vi "SmartSEM Remote API save FIB probe table.vi"(8 "error in":errorcluster, 10 "FIB Probe":string(combo), 11 "ActiveX Container":refnum<k7>(container)) -> (0 "error out":errorcluster, 3 "reference out":refnum<k7>)   [LabVIEW 2018]
uses:
  <vilib>/Utility/file.llb/Write To Spreadsheet File (string).vi
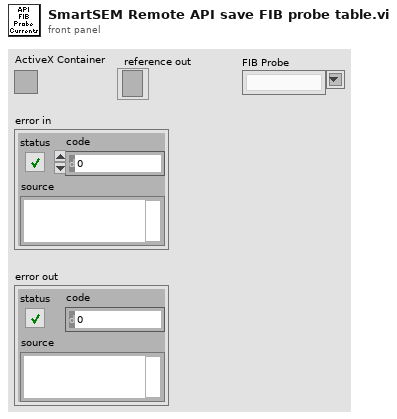
[diagram p1: front panel]
types:
  T1 = cluster{"FIB mode":u8, "FIB focus":sgl, "FIB probe current":sgl, "FIB emission current":sgl, "FIB rotation":sgl, "FIB aperture X":sgl, "FIB aperture Y":sgl, "FIB stig X":sgl, "FIB stig Y":sgl, "FIB beam shift X":sgl, "FIB beam shift Y":sgl}
  T2 = cluster{"Filament (A)":sgl, "Accelerator Target (V)":sgl, "Accelerator Actual (V)":sgl, "Extrator Target (V)":sgl, "Extrator Actual (V)":sgl, "Emission Target (uA)":sgl, "Emission Actual (uA)":sgl, "Suppressor (V)":sgl, "Faraday I (nA)":sgl, "Lens1 Target (V)":sgl, "Lens1 Actual (V)":sgl, "Lens2 Target (V)":sgl, "Lens2 Actual (V)":sgl, "Gun Vac (Torr)":sgl, "Column Vac (Torr)":sgl, "Tip Lifetime (uAhr)":sgl}
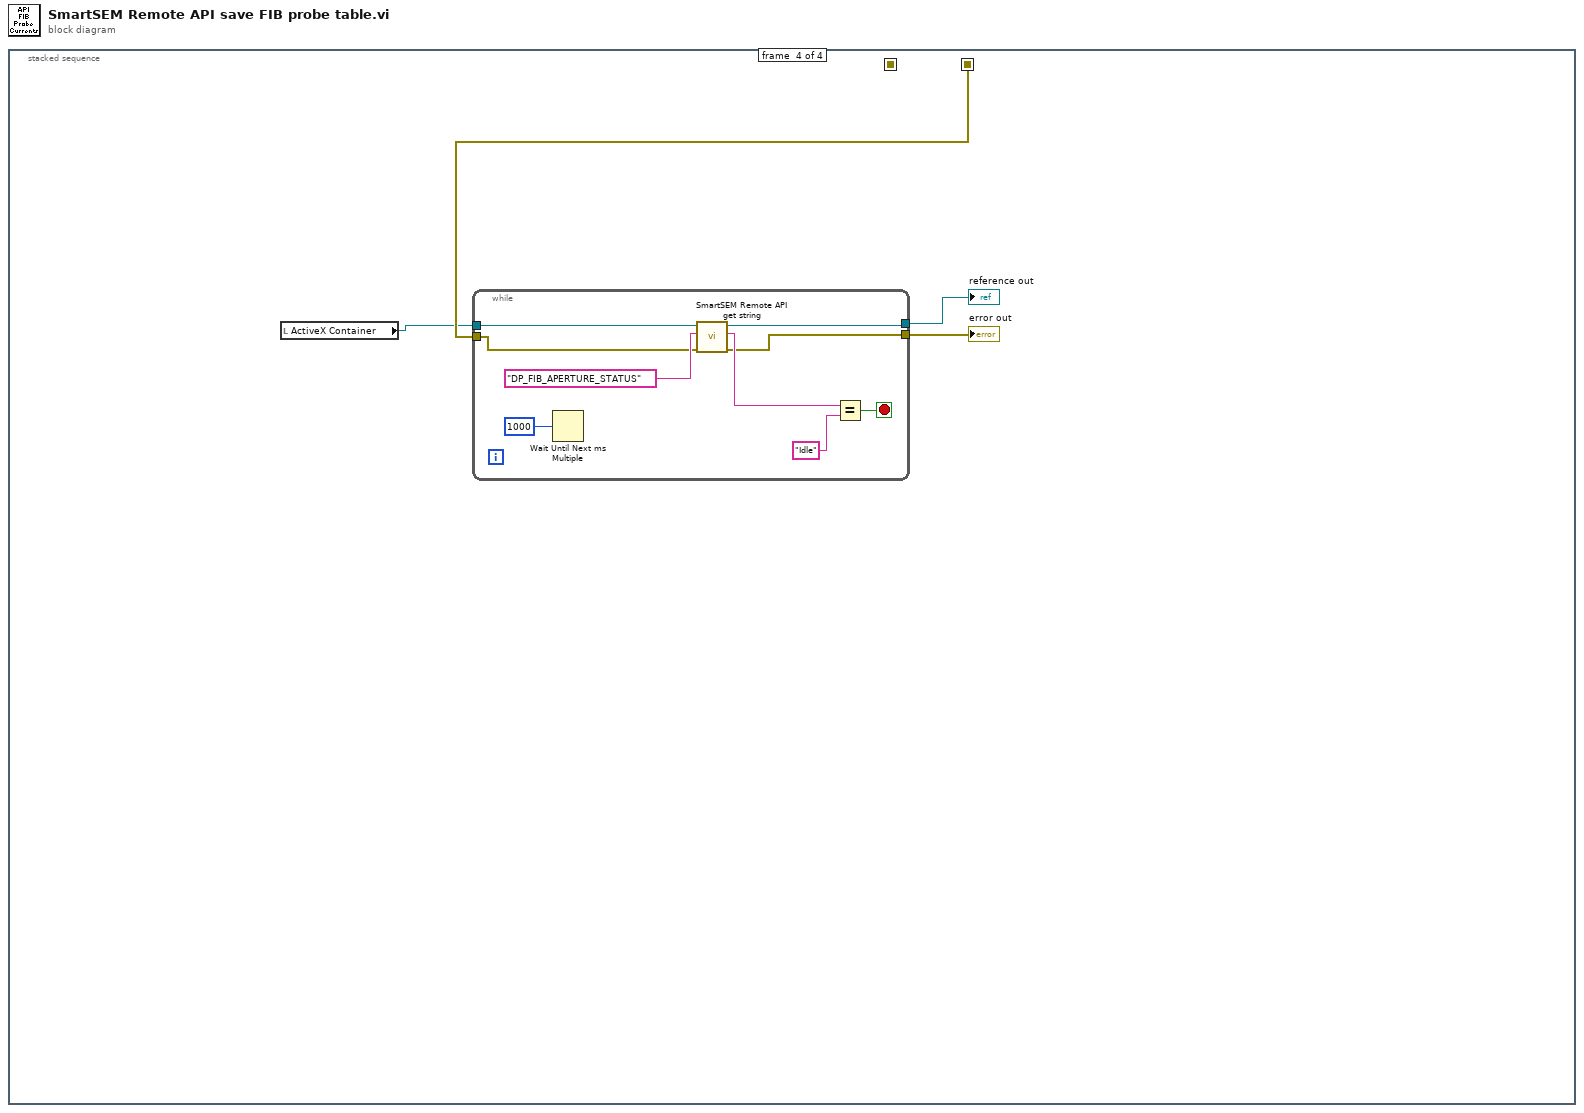
[diagram p0: block diagram]
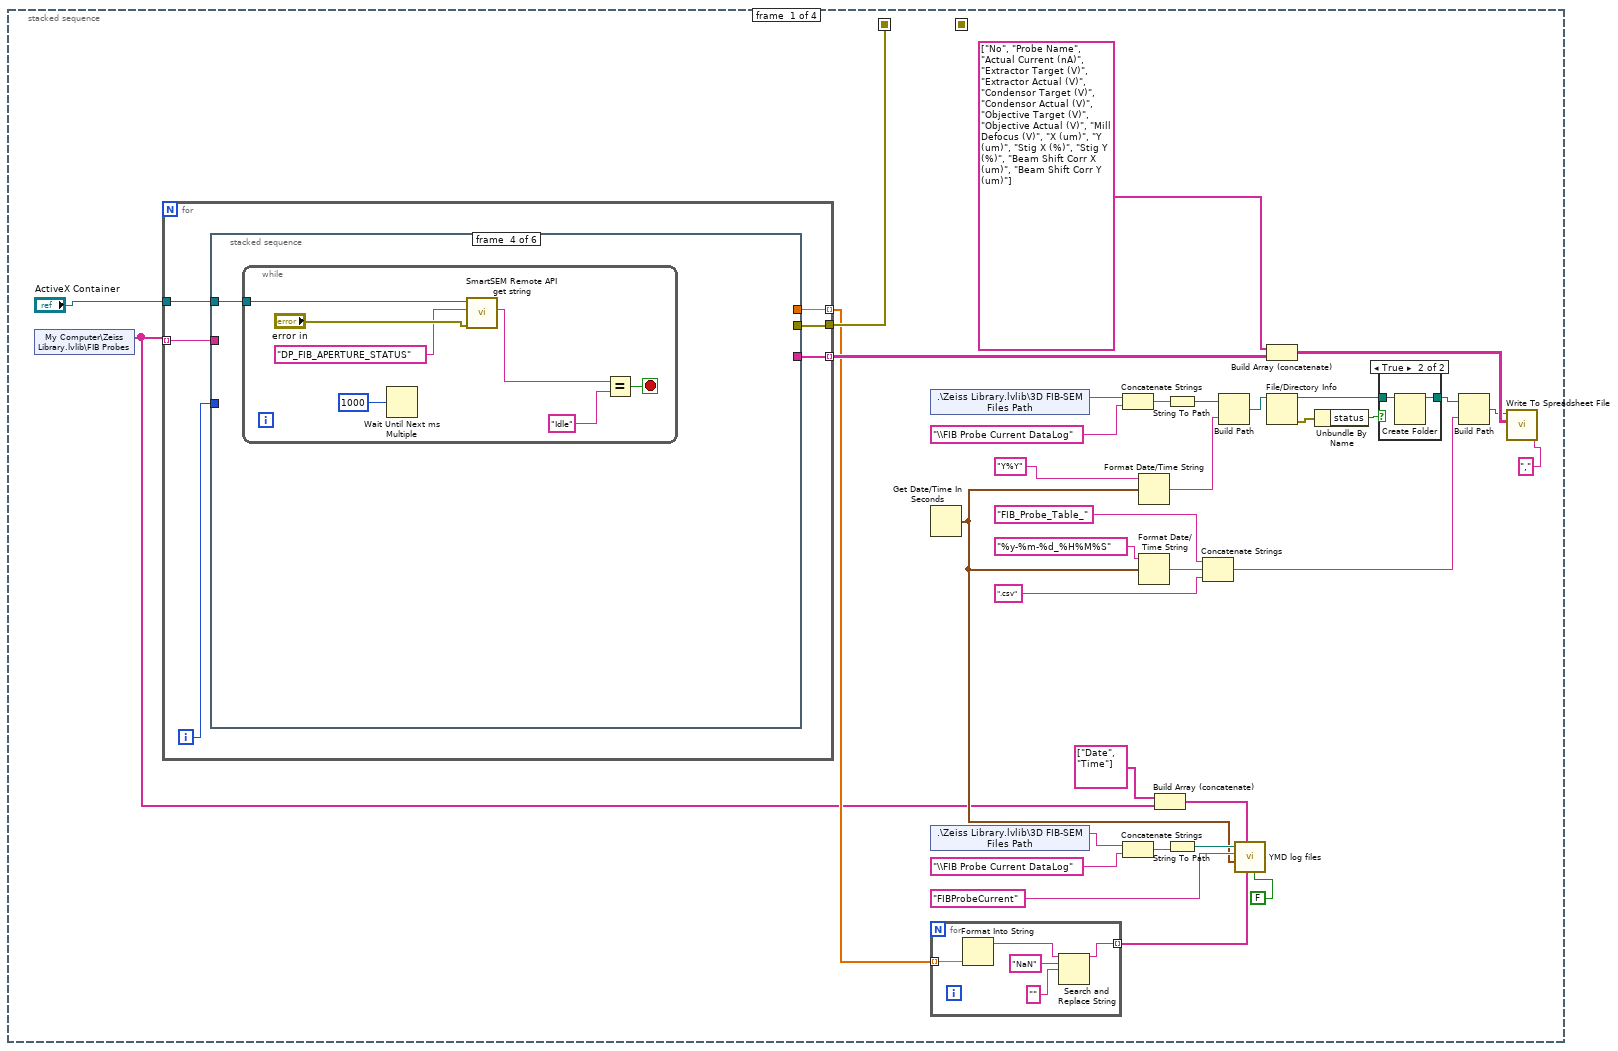
[diagram p2: hidden frame]
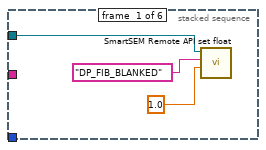
[diagram p4: hidden frame]
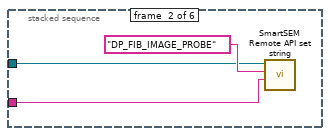
[diagram p5: hidden frame]
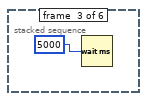
[diagram p6: hidden frame]
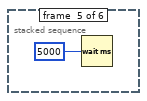
[diagram p7: hidden frame]
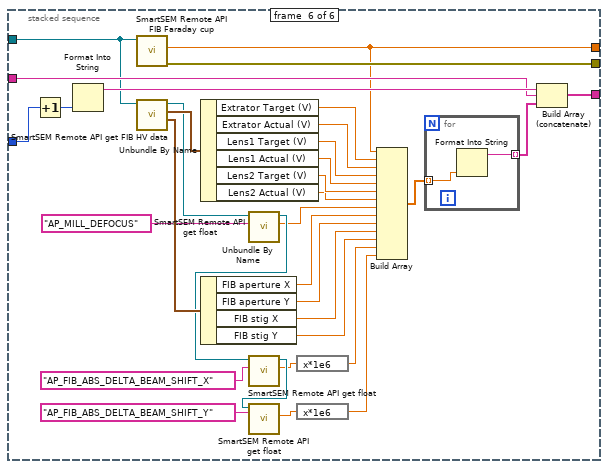
[diagram p8: hidden frame]
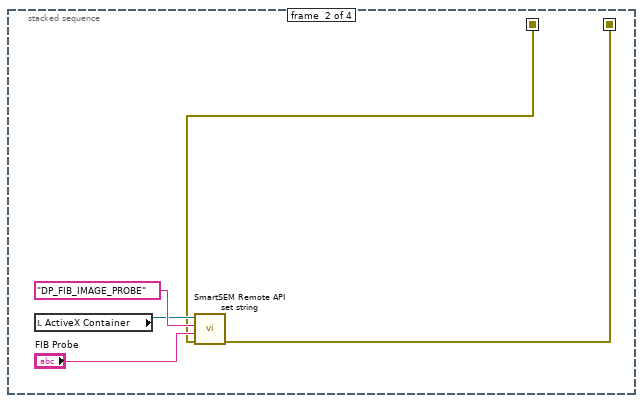
[diagram p9: hidden frame]
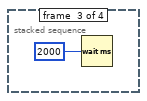
[diagram p10: hidden frame]
diagram:
  n1 = stacked-sequence {
    seq-local: [w25 _ _ _] -> [_ w102 _ _]
    seq-local: [_ w101 _ _] -> [_ _ _ w110]
    frame #0 {
      n2 = shared-variable "My Computer\\Zeiss Library.lvlib\\FIB Probes"() -> (w8:string[])  [unwired: 1 in, 1 out]
      n3 = for {
        tunnel: "ActiveX Container" -> [w49]
        tunnel: [w48] -> w25
        tunnel: w8 -> [w47] mode=indexing
        tunnel: [w45] -> w35 mode=indexing
        tunnel: [w44] -> w10 mode=indexing
        i -> [w46]
        n4 = stacked-sequence {
          tunnel: w47 -> [_ w54 _ _ _ w94]
          tunnel: w49 -> [w50 w53 _ w57 _ w92]
          tunnel: [_ _ _ _ _ w98] -> w48
          tunnel: w46 -> [_ _ _ _ _ w97]
          tunnel: [_ _ _ _ _ w93] -> w45
          tunnel: [_ _ _ _ _ w77] -> w44
          frame #0 {
            n5 = call "SmartSEM Remote API set float.vi"("vValue"=sgl 1.0, "lpszParam"="DP_FIB_BLANKED", "ActiveX Container"=w50) -> ()  [unwired: 7 in, 2 out]
          }
          frame #1 {
            n6 = call "SmartSEM Remote API set string.vi"("vValue"=w54, "lpszParam"="DP_FIB_IMAGE_PROBE", "ActiveX Container"=w53) -> ()  [unwired: 7 in, 2 out]
          }
          frame #2 {
            n7 = Wait (ms)(milliseconds to wait=u32 5000) -> ()  [unwired: 1 out]
          }
          frame #3 {
            n8 = while {
              tunnel: w57 -> [w60]
              stop <- w62 stop-if-true
              n9 = Wait Until Next ms Multiple(millisecond multiple=u32 1000) -> ()  [unwired: 1 out]
              n10 = call "SmartSEM Remote API get string.vi"("error in"="error in", "lpszParam"="DP_FIB_APERTURE_STATUS", "ActiveX Container"=w60) -> ("data"=w58:string)  [unwired: 6 in, 2 out]
              n11 = Equal?(x=w58, y="Idle" ("lpszParam")) -> (x = y?=w62:bool)
            }
          }
          frame #4 {
            n12 = Wait (ms)(milliseconds to wait=u32 5000) -> ()  [unwired: 1 out]
          }
          frame #5 {
            n13 = Increment(x=w97) -> (x+1=w96:i32)
            n14 = Format Into String(w96) -> (resulting string=w95:string)  [unwired: 3 in, 1 out]
            n15 = call "SmartSEM Remote API FIB Faraday cup.vi"("ActiveX Container"=w92) -> ("error out"=w98:errorcluster, "FIB Faraday Cup (nA)"=w77:sgl)  [unwired: 8 in, 1 out]
            n16 = call "SmartSEM Remote API get FIB HV data.vi"("ActiveX Container"=w92) -> ("FIB parameters"=w90:T1, "Capella HV Data Output"=w91:T2, "reference out"=w69:refnum<k7>)  [unwired: 7 in, 1 out]
            n17 = Unbundle By Name(w91) -> ("Extrator Target (V)"=w80:sgl, "Extrator Actual (V)"=w89:sgl, "Lens1 Target (V)"=w88:sgl, "Lens1 Actual (V)"=w79:sgl, "Lens2 Target (V)"=w87:sgl, "Lens2 Actual (V)"=w78:sgl)
            n18 = Unbundle By Name(w90) -> ("FIB aperture X"=w86:sgl, "FIB aperture Y"=w85:sgl, "FIB stig X"=w84:sgl, "FIB stig Y"=w83:sgl)
            n19 = call "SmartSEM Remote API get float.vi"("lpszParam"="AP_MILL_DEFOCUS", "ActiveX Container"=w69) -> ("vValue"=w67:sgl, "reference out"=w68:refnum<k7>)  [unwired: 7 in, 1 out]
            n20 = call "SmartSEM Remote API get float.vi"("lpszParam"="AP_FIB_ABS_DELTA_BEAM_SHIFT_X", "ActiveX Container"=w68) -> ("vValue"=w73:sgl, "reference out"=w74:refnum<k7>)  [unwired: 7 in, 1 out]
            n21 = call "SmartSEM Remote API get float.vi"("lpszParam"="AP_FIB_ABS_DELTA_BEAM_SHIFT_Y", "ActiveX Container"=w74) -> ("vValue"=w71:sgl)  [unwired: 7 in, 2 out]
            n22 = expression code="x*1e6"(w73) -> (w72:sgl)
            n23 = expression code="x*1e6"(w71) -> (w70:sgl)
            n24 = Build Array(w77, w80, w89, w88, w79, w87, w78, w67, w86, w85, w84, w83, w72, w70) -> (w82:sgl[])
            n25 = for {
              tunnel: w82 -> [w100] mode=indexing
              tunnel: [w99] -> w81 mode=indexing
              n26 = Format Into String(w100) -> (resulting string=w99:string)  [unwired: 3 in, 1 out]
            }
            n27 = Build Array (concatenate)(w95, w94, w81) -> (w93:string[])
          }
        }
      }
      n28 = shared-variable ".\\Zeiss Library.lvlib\\3D FIB-SEM Files Path"() -> (w27:string)  [unwired: 1 in, 1 out]
      n29 = Get Date/Time In Seconds() -> (seconds since 1Jan1904=w9:timestamp)
      n30 = shared-variable ".\\Zeiss Library.lvlib\\3D FIB-SEM Files Path"() -> (w14:string)  [unwired: 1 in, 1 out]
      n31 = for {
        tunnel: [w39] -> w15 mode=indexing
        tunnel: w10 -> [w43] mode=indexing
        n32 = Format Into String(w43) -> (resulting string=w40:string)  [unwired: 3 in, 1 out]
        n33 = Search and Replace String(input string=w40, search string="NaN", replace string="" ("replace string (\"\")")) -> (result string=w39:string)  [unwired: 5 in, 3 out]
      }
      n34 = Concatenate Strings(w27, "\\FIB Probe Current DataLog" ("Log file name")) -> (w26:string)
      n35 = Concatenate Strings(w14, "\\FIB Probe Current DataLog" ("Log file name")) -> (w12:string)
      n36 = Format Date/Time String(time format string (%c)="Y%Y", seconds (now)=w9) -> (date/time string=w31:string)  [unwired: 1 out]
      n37 = Format Date/Time String(time format string (%c)="%y-%m-%d_%H%M%S", seconds (now)=w9) -> (date/time string=w22:string)  [unwired: 1 out]
      n38 = Build Array (concatenate)(string[] ["Date", "Time"], w8) -> (w16:string[])
      n39 = String To Path(string=w26) -> (path=w29:path)
      n40 = String To Path(string=w12) -> (path=w11:path)
      n41 = Concatenate Strings("FIB_Probe_Table_" ("time format string (%c)"), w22, ".csv" ("time format string (%c)")) -> (w20:string)
      n42 = Build Path(base path=w29, name or relative path=w31) -> (appended path=w3:path)
      n43 = call "YMD log files.vi"("Day"=FALSE ("Month"), "Input text array"=w15, "Input header array"=w16, "current time"=w9, "Log file name"="FIBProbeCurrent", "Log file path"=w11) -> ()  [unwired: 6 in]
      n44 = Build Array (concatenate)(string[] ["No", "Probe Name", "Actual Current (nA)", "Extractor Target (V)", "Extractor Actual (V)", "Condensor Target (V)", "Condensor Actual (V)", "Objective Target (V)", "Objective Actual (V)", "Mill Defocus (V)", "X (um)", "Y (um)", "Stig X (%)", "Stig Y (%)", "Beam Shift Corr X (um)", "Beam Shift Corr Y (um)"], w35) -> (w33:string[][])
      n45 = File/Directory Info(path=w3) -> (path out=w6:path, error out=w5:errorcluster)  [unwired: 1 in, 5 out]
      n46 = Unbundle By Name(w5) -> ("status"=w7:bool)
      n47 = case shown="True" w7 {
        tunnel: w6 -> [w36 w37]
        tunnel: [w36 w38] -> w2
        frame False {
        }
        frame True {
          n48 = Create Folder(path (use dialog)=w37) -> (created path=w38:path)  [unwired: 2 in, 2 out]
        }
      }
      n49 = Build Path(base path=w2, name or relative path=w20) -> (appended path=w4:path)
      n50 = call-poly <vilib>:"Write To Spreadsheet File.vi"("delimiter (\\t)"="," ("delimiter (\\t)"), "2D data"=w33, "file path (dialog if empty)"=w4) -> ()  [unwired: 5 in, 1 out]
    }
    frame #1 {
      n51 = local read "ActiveX Container"() -> (w103:refnum<k7>)
      n52 = call "SmartSEM Remote API set string.vi"("error in"=w102, "vValue"="FIB Probe", "lpszParam"="DP_FIB_IMAGE_PROBE", "ActiveX Container"=w103) -> ("error out"=w101:errorcluster)  [unwired: 6 in, 1 out]
    }
    frame #2 {
      n53 = Wait (ms)(milliseconds to wait=u32 2000) -> ()  [unwired: 1 out]
    }
    frame #3 {
      n54 = local read "ActiveX Container"() -> (w107:refnum<k7>)
      n55 = while {
        tunnel: w107 -> [w116]
        tunnel: w110 -> [w113]
        tunnel: [w111] -> w109
        tunnel: [w112] -> w108
        stop <- w117 stop-if-true
        n56 = Wait Until Next ms Multiple(millisecond multiple=u32 1000) -> ()  [unwired: 1 out]
        n57 = call "SmartSEM Remote API get string.vi"("error in"=w113, "lpszParam"="DP_FIB_APERTURE_STATUS", "ActiveX Container"=w116) -> ("error out"=w111:errorcluster, "data"=w114:string, "reference out"=w112:refnum<k7>)  [unwired: 6 in]
        n58 = Equal?(x=w114, y="Idle" ("lpszParam")) -> (x = y?=w117:bool)
      }
      "error out" <- w109
      "reference out" <- w108
    }
  }
